vi "Read Instrument Identifiers.vi"(7 "Unit Address (1)":u8=1, 8 "error in (no error)":errorcluster, 11 "VISA resource name":refnum<visa-resource-name>) -> (0 "error out":errorcluster, 1 "Company ID":u16, 2 "Instrument Version Number":u16 format="%x", 3 "VISA resource name out":refnum<visa-resource-name>, 4 "Customer Defined ID (0)":u16, 5 "Instrument Identity":i16 format="%x")   [LabVIEW 2014, in "Eurotherm 35xx Series.lvlib"]
doc: "This VI returns Instrument Identifiers."
uses:
  <instrlib>/Eurotherm 35xx Series/Eurotherm 35xx Series.lvlib
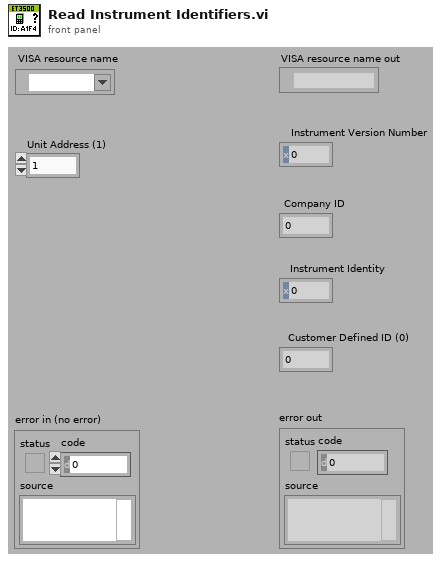
[diagram p1: front panel]
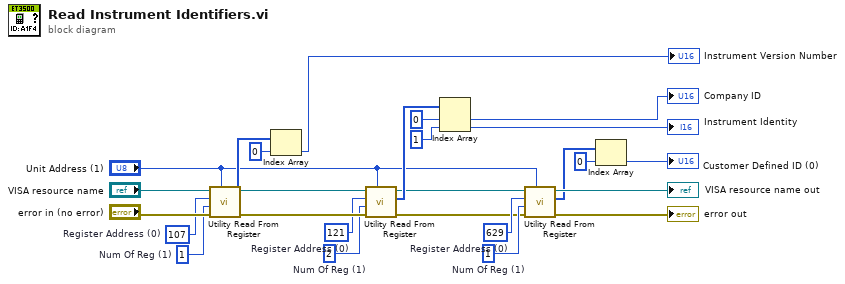
[diagram p0: block diagram]
diagram:
  w11 = u16 629  # Register Address (0)
  w10 = u16 1  # Num Of Reg (1)
  w16 = u16 121  # Register Address (0)
  w17 = u16 107  # Register Address (0)
  w18 = u16 2  # Num Of Reg (1)
  w24 = u16 1  # Num Of Reg (1)
  n1 = call <instrlib>:"Utility Read From Register.vi"("Unit Address (1)"="Unit Address (1)", "error in (no error)"="error in (no error)", "Num Of Reg (1)"=w24, "Register Address (0)"=w17, "VISA resource name"="VISA resource name") -> ("error out"=w19:errorcluster, "Data"=w23:i16[], "VISA resource name out"=w20:refnum<visa-resource-name>)  [unwired: 4 in]
  n2 = Index Array(array=w23, index=0) -> (element=→"Instrument Version Number":i16)
  n3 = call <instrlib>:"Utility Read From Register.vi"("Unit Address (1)"="Unit Address (1)", "error in (no error)"=w19, "Num Of Reg (1)"=w18, "Register Address (0)"=w16, "VISA resource name"=w20) -> ("error out"=w6:errorcluster, "Data"=w13:i16[], "VISA resource name out"=w7:refnum<visa-resource-name>)  [unwired: 4 in]
  n4 = Index Array(array=w13, index #1=0 ("index"), index #2=1 ("index")) -> (element #1=→"Company ID":i16, element #2=→"Instrument Identity":i16)
  n5 = call <instrlib>:"Utility Read From Register.vi"("Unit Address (1)"="Unit Address (1)", "error in (no error)"=w6, "Num Of Reg (1)"=w10, "Register Address (0)"=w11, "VISA resource name"=w7) -> ("error out"=→"error out":errorcluster, "Data"=w4:i16[], "VISA resource name out"=→"VISA resource name out":refnum<visa-resource-name>)  [unwired: 4 in]
  n6 = Index Array(array=w4, index=0) -> (element=→"Customer Defined ID (0)":i16)
